vi "niRFUtil WFM Average (real scalar).vi"(0 "Data In":sgl format="%.2f", 5 "Average Mode":enum16{"Exponential", "Repeat"}(ring), 7 "Average Method":T1, 12 "Reset?":bool=TRUE, 13 "Initialize?":bool=TRUE) -> (4 "Average Out":sgl format="%.2f")   [LabVIEW 2015, in "niRFUtil.lvlib"]
doc: "(c) Copyright 2006, National Instruments, Inc. This VI may not be duplicated, sold, or distributed without written consent from National Instruments."
uses:
  niRFUtil.lvlib
  Includes/niRFUtil INC Average Methods.ctl
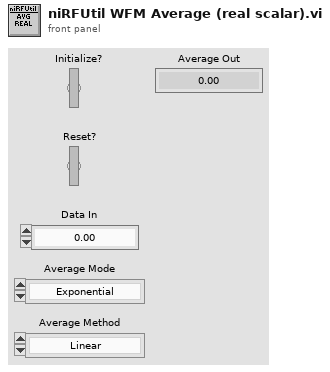
[diagram p1: front panel]
types:
  T1 = typedef "niRFUtil.lvlib/niRFUtil INC Average Methods.ctl" = enum16{"Linear", "Log", "Root", "Max", "Min", "MinMax"}
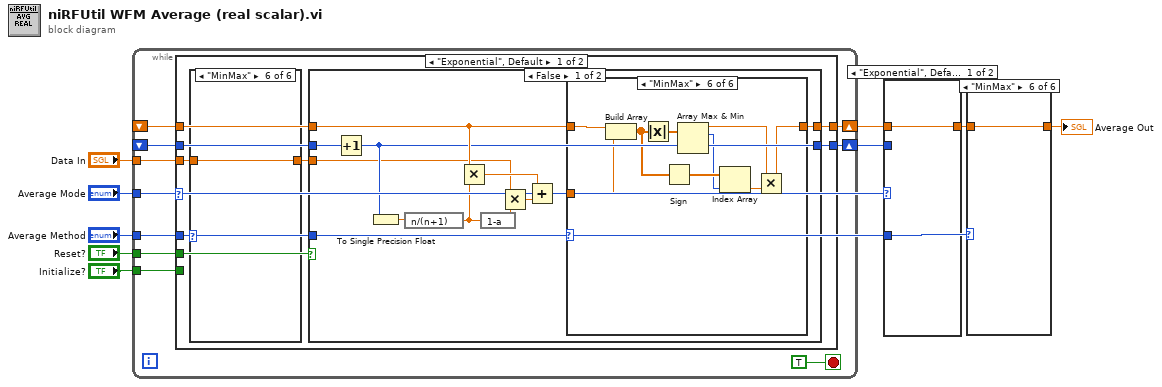
[diagram p0: block diagram]
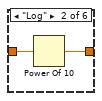
[diagram p3: hidden frame]
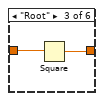
[diagram p4: hidden frame]
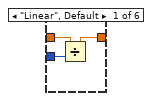
[diagram p8: hidden frame]
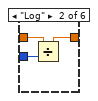
[diagram p9: hidden frame]
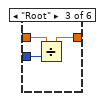
[diagram p10: hidden frame]
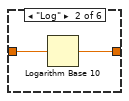
[diagram p14: hidden frame]
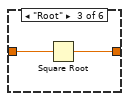
[diagram p15: hidden frame]
diagram:
  n1 = while {
    shift-right: [w16] -> w7
    shift-left: _ -> [w13]
    tunnel: "Average Mode" -> [w18]
    tunnel: "Reset?" -> [w17]
    tunnel: "Data In" -> [w15]
    shift-right: [w14] -> w5
    shift-left: _ -> [w12]
    tunnel: "Average Method" -> [w11]
    tunnel: "Initialize?" -> [w10]
    stop <- TRUE stop-if-true
    n2 = case shown="\"Exponential\", Default" w18 {
      tunnel: w17 -> [w24 _]
      tunnel: [w27 w75] -> w16
      tunnel: w15 -> [w22 w70]
      tunnel: [w23 w72] -> w14
      tunnel: w13 -> [w26 w74]
      tunnel: w12 -> [w25 w73]
      tunnel: w11 -> [w20 w68]
      tunnel: w10 -> [_ w71]
      frame "Exponential", Default {
        n3 = case shown="\"MinMax\"" w20 {
          tunnel: w22 -> [w28 w30 w32 w33 w34 w35]
          tunnel: [w28 w29 w31 w33 w34 w35] -> w21
          frame "Linear", Default {
          }
          frame "Log" {
            n4 = Logarithm Base 10(1:w30) -> (0:w29:sgl)
          }
          frame "Root" {
            n5 = Square Root(x=w32) -> (sqrt(x)=w31:sgl)
          }
          frame "Max" {
          }
          frame "Min" {
          }
          frame "MinMax" {
          }
        }
        n6 = case shown="False" w24 {
          tunnel: w21 -> [w36 w66]
          tunnel: [w42 w66] -> w27
          tunnel: w26 -> [w40 _]
          tunnel: w25 -> [w39 _]
          tunnel: [w38 1] -> w23
          tunnel: w20 -> [w37 _]
          frame False {
            n7 = Increment(x=w39) -> (x+1=w38:i32)
            n8 = To Single Precision Float(number=w38) -> (single precision float=w47:sgl)
            n9 = expression code="n/(n+1)"(w47) -> (w46:sgl)
            n10 = Multiply(x=w40, y=w46) -> (x*y=w43:sgl)
            n11 = expression code="1-a"(w46) -> (w45:sgl)
            n12 = Multiply(x=w36, y=w45) -> (x*y=w44:sgl)
            n13 = Add(x=w43, y=w44) -> (x+y=w41:sgl)
            n14 = case shown="\"MinMax\"" w37 {
              tunnel: [w48 w49 w50 w51 w54 w63] -> w42
              tunnel: w41 -> [w48 w49 w50 w52 w55 w64]
              tunnel: w40 -> [_ _ _ w53 w56 w65]
              frame "Linear", Default {
              }
              frame "Log" {
              }
              frame "Root" {
              }
              frame "Max" {
                n15 = Max & Min(x=w53, y=w52) -> (max(x,y)=w51:sgl)  [unwired: 1 out]
              }
              frame "Min" {
                n16 = Max & Min(x=w56, y=w55) -> (min(x,y)=w54:sgl)  [unwired: 1 out]
              }
              frame "MinMax" {
                n17 = Build Array(w65, w64) -> (w62:sgl[])
                n18 = Absolute Value(x=w62) -> (abs(x)=w59:sgl[])
                n19 = Sign(1:w62) -> (0:w61:sgl[])
                n20 = Array Max & Min(array=w59) -> (max value=w58:sgl, max index (indices)=w57:i32)  [unwired: 2 out]
                n21 = Index Array(array=w61, index=w57) -> (element=w60:sgl)
                n22 = Multiply(x=w58, y=w60) -> (x*y=w63:sgl)
              }
            }
          }
          frame True {
          }
        }
      }
      frame "Repeat" {
        n23 = case shown="\"MinMax\"" w68 {
          tunnel: w70 -> [w76 w78 w80 w81 w82 w83]
          tunnel: [w76 w77 w79 w81 w82 w83] -> w69
          frame "Linear", Default {
          }
          frame "Log" {
            n24 = Logarithm Base 10(1:w78) -> (0:w77:sgl)
          }
          frame "Root" {
            n25 = Square Root(x=w80) -> (sqrt(x)=w79:sgl)
          }
          frame "Max" {
          }
          frame "Min" {
          }
          frame "MinMax" {
          }
        }
        n26 = case shown="False" w71 {
          tunnel: w69 -> [w84 w114]
          tunnel: [w89 w114] -> w75
          tunnel: w74 -> [w88 _]
          tunnel: w73 -> [w87 _]
          tunnel: [w86 1] -> w72
          tunnel: w68 -> [w85 _]
          frame False {
            n27 = Increment(x=w87) -> (x+1=w86:i32)
            n28 = case shown="\"MinMax\"" w85 {
              tunnel: [w90 w93 w96 w99 w102 w111] -> w89
              tunnel: w88 -> [w91 w94 w97 w101 w104 w113]
              tunnel: w84 -> [w92 w95 w98 w100 w103 w112]
              frame "Linear", Default {
                n29 = Add(x=w91, y=w92) -> (x+y=w90:sgl)
              }
              frame "Log" {
                n30 = Add(x=w94, y=w95) -> (x+y=w93:sgl)
              }
              frame "Root" {
                n31 = Add(x=w97, y=w98) -> (x+y=w96:sgl)
              }
              frame "Max" {
                n32 = Max & Min(x=w101, y=w100) -> (max(x,y)=w99:sgl)  [unwired: 1 out]
              }
              frame "Min" {
                n33 = Max & Min(x=w104, y=w103) -> (min(x,y)=w102:sgl)  [unwired: 1 out]
              }
              frame "MinMax" {
                n34 = Build Array(w113, w112) -> (w110:sgl[])
                n35 = Absolute Value(x=w110) -> (abs(x)=w107:sgl[])
                n36 = Sign(1:w110) -> (0:w109:sgl[])
                n37 = Array Max & Min(array=w107) -> (max value=w106:sgl, max index (indices)=w105:i32)  [unwired: 2 out]
                n38 = Index Array(array=w109, index=w105) -> (element=w108:sgl)
                n39 = Multiply(x=w106, y=w108) -> (x*y=w111:sgl)
              }
            }
          }
          frame True {
          }
        }
      }
    }
  }
  n40 = case shown="\"Exponential\", Default" "Average Mode" {
    tunnel: [w116 w118] -> w2
    tunnel: w7 -> [w116 w119]
    tunnel: w5 -> [_ w120]
    tunnel: "Average Method" -> [_ w117]
    frame "Exponential", Default {
    }
    frame "Repeat" {
      n41 = case shown="\"MinMax\"" w117 {
        tunnel: w120 -> [w123 w126 w129 _ _ _]
        tunnel: w119 -> [w122 w125 w128 w130 w131 w132]
        tunnel: [w121 w124 w127 w130 w131 w132] -> w118
        frame "Linear", Default {
          n42 = Divide(x=w122, y=w123) -> (x/y=w121:sgl)
        }
        frame "Log" {
          n43 = Divide(x=w125, y=w126) -> (x/y=w124:sgl)
        }
        frame "Root" {
          n44 = Divide(x=w128, y=w129) -> (x/y=w127:sgl)
        }
        frame "Max" {
        }
        frame "Min" {
        }
        frame "MinMax" {
        }
      }
    }
  }
  n45 = case shown="\"MinMax\"" "Average Method" {
    tunnel: w2 -> [w133 w135 w137 w138 w139 w140]
    tunnel: [w133 w134 w136 w138 w139 w140] -> w1
    frame "Linear", Default {
    }
    frame "Log" {
      n46 = Power Of 10(x=w135) -> (10^x=w134:sgl)
    }
    frame "Root" {
      n47 = Square(x=w137) -> (x^2=w136:sgl)
    }
    frame "Max" {
    }
    frame "Min" {
    }
    frame "MinMax" {
    }
  }
  "Average Out" <- w1
